vi "process_nested.vi"(11 "RESP3 Parser in":refnum<class "RESP3 Parser.lvclass">) -> (0 "error out":errorcluster, 1 "RESP3 Value":variant, 2 "value ready?":bool, 3 "RESP3 Parser out":refnum<class "RESP3 Parser.lvclass">)   [LabVIEW 2019, in "RESP3.lvlib" / "RESP3 Parser.lvclass"]
uses:
  RESP3 Parser.lvclass
  RESP3 Parser.lvclass/RESP3 Parser.ctl
  RESP3.lvlib
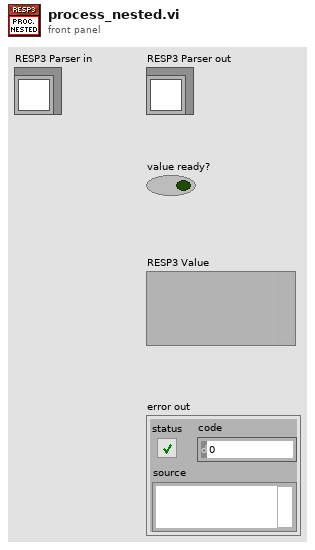
[diagram p1: front panel]
types:
  T1 = typedef "RESP3.lvlib/RESP3 Type.ctl" = enum8{"<0x00>", "<0x01>", "<0x02>", "<0x03>", "<0x04>", "<0x05>", "<0x06>", "<0x07>", "<0x08>", "<0x09>", "<0x0A>", "<0x0B>", "<0x0C>", "<0x0D>", "<0x0E>", "<0x0F>", "<0x10>", "<0x11>", "<0x12>", "<0x13>", "<0x14>", "<0x15>", "<0x16>", "<0x17>", "<0x18>", "<0x19>", "<0x1A>", "<0x1B>", "<0x1C>", "<0x1D>", "<0x1E>", "<0x1F>", "\" \"", "BLOB ERROR", "\"\"\"", "BOOLEAN", "BLOB", "MAP", "\"&\"", "\"'\"", "BIG NUMBER", "\")\"", "ARRAY", "STRING", "DOUBLE", "ERROR", "END", "\"/\"", "\"0\"", "\"1\"", "\"2\"", "\"3\"", "\"4\"", "\"5\"", "\"6\"", "\"7\"", "\"8\"", "\"9\"", "INTEGER", "STREAM", "\"<\"", "VERBATIM STRING", "PUSH", "\"?\"", "\"@\"", "\"A\"", "\"B\"", "\"C\"", "\"D\"", "\"E\"", "\"F\"", "\"G\"", "\"H\"", "\"I\"", "\"J\"", "\"K\"", "\"L\"", "\"M\"", "\"N\"", "\"O\"", "\"P\"", "\"Q\"", "\"R\"", "\"S\"", "\"T\"", "\"U\"", "\"V\"", "\"W\"", "\"X\"", "\"Y\"", "\"Z\"", "\"[\"", "\"\\\"", "\"]\"", "\"^\"", "NULL", "\"`\"", "\"a\"", "\"b\"", "\"c\"", "\"d\"", "\"e\"", "\"f\"", "\"g\"", "\"h\"", "\"i\"", "\"j\"", "\"k\"", "\"l\"", "\"m\"", "\"n\"", "\"o\"", "\"p\"", "\"q\"", "\"r\"", "\"s\"", "\"t\"", "\"u\"", "\"v\"", "\"w\"", "\"x\"", "\"y\"", "\"z\"", "\"{\"", "ATTRIBUTES", "\"}\"", "SET", "<0x7F>", "<0x80>", "<0x81>", "<0x82>", "<0x83>", "<0x84>", "<0x85>", "<0x86>", "<0x87>", "<0x88>", "<0x89>", "<0x8A>", "<0x8B>", "<0x8C>", "<0x8D>", "<0x8E>", "<0x8F>", "<0x90>", "<0x91>", "<0x92>", "<0x93>", "<0x94>", "<0x95>", "<0x96>", "<0x97>", "<0x98>", "<0x99>", "<0x9A>", "<0x9B>", "<0x9C>", "<0x9D>", "<0x9E>", "<0x9F>", "<0xA0>", "<0xA1>", "<0xA2>", "<0xA3>", "<0xA4>", "<0xA5>", "<0xA6>", "<0xA7>", "<0xA8>", "<0xA9>", "<0xAA>", "<0xAB>", "<0xAC>", "<0xAD>", "<0xAE>", "<0xAF>", "<0xB0>", "<0xB1>", "<0xB2>", "<0xB3>", "<0xB4>", "<0xB5>", "<0xB6>", "<0xB7>", "<0xB8>", "<0xB9>", "<0xBA>", "<0xBB>", "<0xBC>", "<0xBD>", "<0xBE>", "<0xBF>", "<0xC0>", "<0xC1>", "<0xC2>", "<0xC3>", "<0xC4>", "<0xC5>", "<0xC6>", "<0xC7>", "<0xC8>", "<0xC9>", "<0xCA>", "<0xCB>", "<0xCC>", "<0xCD>", "<0xCE>", "<0xCF>", "<0xD0>", "<0xD1>", "<0xD2>", "<0xD3>", "<0xD4>", "<0xD5>", "<0xD6>", "<0xD7>", "<0xD8>", "<0xD9>", "<0xDA>", "<0xDB>", "<0xDC>", "<0xDD>", "<0xDE>", "<0xDF>", "<0xE0>", "<0xE1>", "<0xE2>", "<0xE3>", "<0xE4>", "<0xE5>", "<0xE6>", "<0xE7>", "<0xE8>", "<0xE9>", "<0xEA>", "<0xEB>", "<0xEC>", "<0xED>", "<0xEE>", "<0xEF>", "<0xF0>", "<0xF1>", "<0xF2>", "<0xF3>", "<0xF4>", "<0xF5>", "<0xF6>", "<0xF7>", "<0xF8>", "<0xF9>", "<0xFA>", "<0xFB>", "<0xFC>", "<0xFD>", "<0xFE>"}
  T2 = cluster{"index":i32, "remaining elements":i32, "nest type":T1}[]
  T3 = cluster{"index":i32, "remaining elements":i32, "nest type":T1}
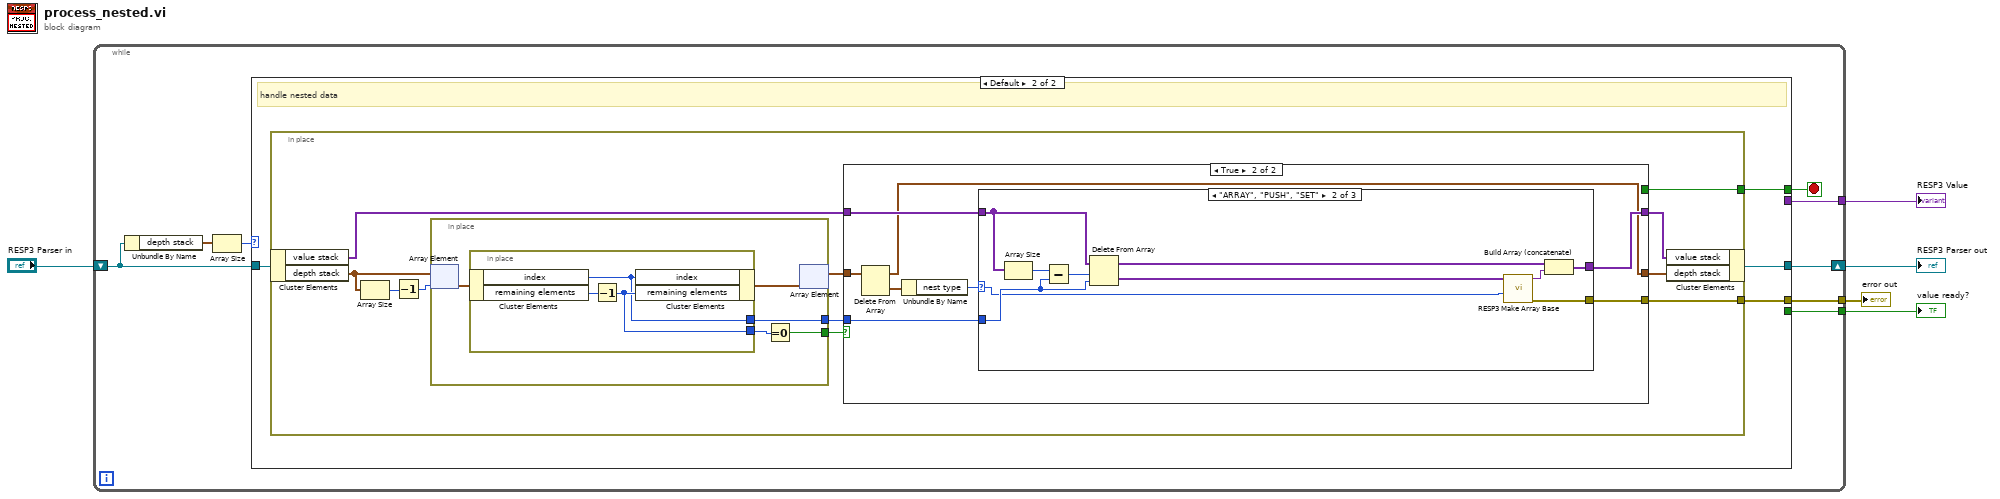
[diagram p0: block diagram]
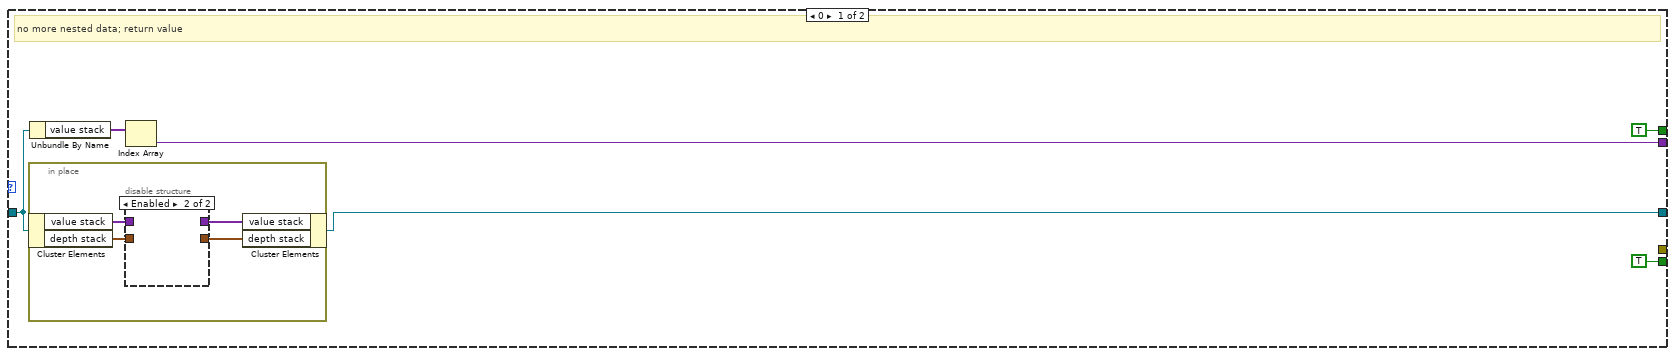
[diagram p2: hidden frame]
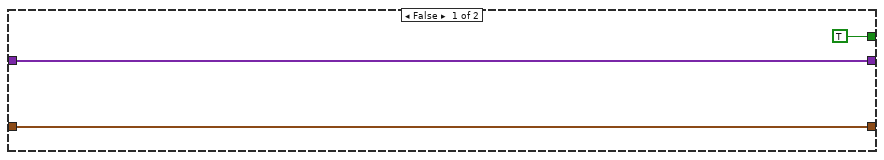
[diagram p4: hidden frame]
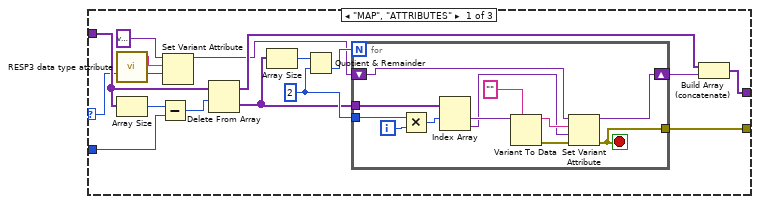
[diagram p5: hidden frame]
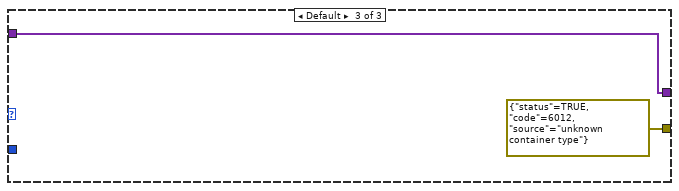
[diagram p6: hidden frame]
diagram:
  n1 = while {
    shift-right: [w10] -> w3
    shift-left: "RESP3 Parser in" -> [w11]
    tunnel: [w9] -> w4
    tunnel: [w8] -> w5
    tunnel: [w6] -> w1
    stop <- w7 stop-if-true
    n2 = Unbundle By Name(w11) -> ("depth stack"=w13:T2)
    n3 = Array Size(array=w13) -> (size(s)=w12:i32)
    n4 = case shown="Default" w12 {
      tunnel: w11 -> [w18 w29]
      tunnel: [w17 w28] -> w10
      tunnel: [w16 _] -> w9
      tunnel: [TRUE _] -> w8
      tunnel: [TRUE w27] -> w7
      tunnel: [_ w26] -> w6
      frame 0 {
        # "no more nested data; return value"
        n5 = in-place {
          n6 = in-place-cluster #1(w18) -> ("value stack"=w22:variant[], "depth stack"=w20:T2)
          n7 = disable-structure shown="Enabled" {
            disable-tunnel: [w25 _] -> w23
            disable-tunnel: w22 -> [w25 _]
            disable-tunnel: [w24 _] -> w21
            disable-tunnel: w20 -> [w24 _]
            frame Disabled {
            }
            frame Enabled {
            }
          }
          n8 = in-place-cluster #1("value stack"=w23, "depth stack"=w21) -> (w17:refnum<class "RESP3 Parser.lvclass">)
        }
        n9 = Unbundle By Name(w18) -> ("value stack"=w19:variant[])
        n10 = Index Array(array=w19) -> (element=w16:variant)  [unwired: 1 in]
      }
      frame Default {
        # "handle nested data"
        n11 = in-place {
          in-place-border: [w31] -> w27
          in-place-border: [w30] -> w26
          n12 = in-place-cluster #2(w29) -> ("value stack"=w37:variant[], "depth stack"=w40:T2)
          n13 = Array Size(array=w40) -> (size(s)=w39:i32)
          n14 = Decrement(x=w39) -> (x-1=w38:i32)
          n15 = in-place {
            in-place-border: [w93] -> w35
            in-place-border: [w92] -> w36
            n16 = in-place-array #3(w40, w38) -> (w96:T3)
            n17 = in-place {
              in-place-border: [w98] -> w95
              in-place-border: [w97] -> w93
              n18 = in-place-cluster #4(w96) -> ("index"=w97:i32, "remaining elements"=w99:i32)
              n19 = Decrement(x=w99) -> (x-1=w98:i32)
              n20 = in-place-cluster #4("index"=w97, "remaining elements"=w98) -> (w94:T3)
            }
            n21 = Equal To 0?(x=w95) -> (x = 0?=w92:bool)
            n22 = in-place-array #3(w94) -> (w33:T2)  [unwired: 1 out]
          }
          n23 = case shown="True" w36 {
            tunnel: w37 -> [w43 w51]
            tunnel: w35 -> [_ w50]
            tunnel: [w43 w49] -> w34
            tunnel: [w42 w47] -> w32
            tunnel: w33 -> [w42 w48]
            tunnel: [TRUE _] -> w31
            tunnel: [_ w44] -> w30
            frame False {
            }
            frame True {
              n24 = Delete From Array(array=w48) -> (deleted portion=w46:T3, array with subset deleted=w47:T2)  [unwired: 2 in]
              n25 = Unbundle By Name(w46) -> ("nest type"=w45:T1)
              n26 = case shown="\"ARRAY\", \"PUSH\", \"SET\"" w45 {
                selector: w45 -> [w56 w81 _]
                tunnel: w51 -> [w64 w89 w91]
                tunnel: w50 -> [w52 w87 _]
                tunnel: [w63 w82 w91] -> w49
                tunnel: [w53 w80 errorcluster {"status"=TRUE, "code"=6012, "source"="unknown container type"} ("error out")] -> w44
                frame "MAP", "ATTRIBUTES" {
                  w60 = 2 ("y")
                  n27 = call "RESP3 data type attribute.vi"() -> ("dt attribute"=w57:string)  [unwired: 5 in]
                  n28 = Array Size(array=w64) -> (size(s)=w67:i32)
                  n29 = Subtract(x=w67, y=w52) -> (x-y=w66:i32)
                  n30 = Set Variant Attribute(Variant=variant, name=w57, value=w56) -> (Variant out=w55:variant)  [unwired: 1 in, 2 out]
                  n31 = Delete From Array(array=w64, length=w66) -> (deleted portion=w59:variant[], array with subset deleted=w65:variant[])  [unwired: 1 in]
                  n32 = Array Size(array=w59) -> (size(s)=w62:i32)
                  n33 = Quotient & Remainder(x=w62, y=w60) -> (floor(x/y)=w61:i32)  [unwired: 1 out]
                  n34 = for {
                    N: w61 -> [_]
                    tunnel: w60 -> [w78]
                    tunnel: w59 -> [w77]
                    shift-right: [w70] -> w54
                    shift-left: w55 -> [w73]
                    tunnel: [w68] -> w53
                    i -> [w79]
                    stop <- w68 stop-if-true
                    n35 = Multiply(x=w78, y=w79) -> (x*y=w76:i32)
                    n36 = Index Array(array=w77, index #1=w76) -> (element #1=w74:variant, element #2=w71:variant)  [unwired: 1 in]
                    n37 = Variant To Data(type="", Variant=w74) -> (data=w72:string, error out=w69:errorcluster)  [unwired: 1 in]
                    n38 = Set Variant Attribute(Variant=w73, name=w72, value=w71, error in=w69) -> (Variant out=w70:variant, error out=w68:errorcluster)  [unwired: 1 out]
                  }
                  n39 = Build Array (concatenate)(w65, w54) -> (w63:variant[])
                }
                frame "ARRAY", "PUSH", "SET" {
                  n40 = Array Size(array=w89) -> (size(s)=w88:i32)
                  n41 = Subtract(x=w88, y=w87) -> (x-y=w86:i32)
                  n42 = Delete From Array(array=w89, length=w86, index=w87) -> (deleted portion=w85:variant[], array with subset deleted=w84:variant[])
                  n43 = call "RESP3 Make Array Base.vi"("RESP3 Type"=w81, "RESP3 Values in"=w85) -> ("error out"=w80:errorcluster, "RESP3 Value out"=w83:variant)  [unwired: 8 in]
                  n44 = Build Array (concatenate)(w84, w83) -> (w82:variant[])
                }
                frame Default {
                }
              }
            }
          }
          n45 = in-place-cluster #2("value stack"=w34, "depth stack"=w32) -> (w28:refnum<class "RESP3 Parser.lvclass">)
        }
      }
    }
  }
  "value ready?" <- w5
  "RESP3 Value" <- w4
  "RESP3 Parser out" <- w3
  "error out" <- w1
